vi "_readArray.vi"(8 "error in (no error)":errorcluster, 11 "JSONParser in":refnum<class "tJSONParser.lvclass">) -> (0 "error out":errorcluster, 2 "tBSONArray Out":refnum<class "tBSONArray.lvclass">, 3 "JSONParser out":refnum<class "tJSONParser.lvclass">)   [LabVIEW 2013, in "JSON.lvlib" / "tJSONParser.lvclass"]
doc: "Reads and validates an array value from a string : value pair. An error is returned if a comma is not followed by an array element."
uses:
  tJSONParser.lvclass
  BSON/BSONElements/tBSONArray/tBSONArray.lvclass
  BSON/tBSONElement/tBSONElement.lvclass
  tJSONParser.lvclass/tJSONParser.ctl
  _tokenType.ctl
  _error.ctl
  BSON/BSONElements/tBSONArray/setValue.vi
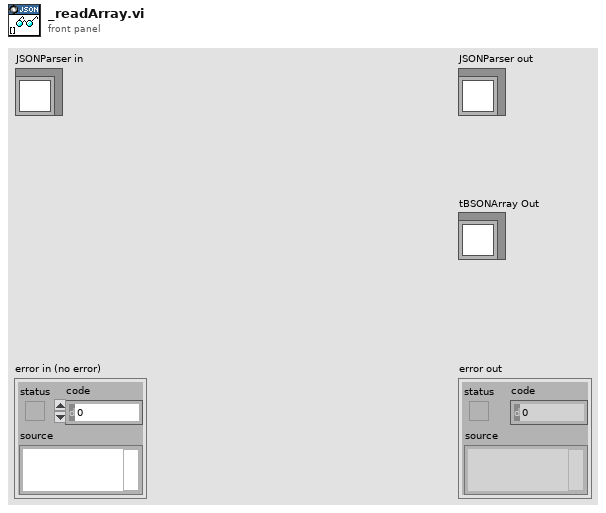
[diagram p1: front panel]
types:
  T1 = typedef "JSON.lvlib/tJSONParser.lvclass/_tokenType.ctl" = enum16{"Object Begin", "Object End", "Array Begin", "Array End", "String Delimeter", "Forward Slash", "Number", "Boolean", "Null", "Object Or Array Separator", "Pair Separator", "End Of File", "Asterisk", "Backward Slash", "Other"}
  T2 = typedef "JSON.lvlib/tJSONParser.lvclass/_error.ctl" = enum16{"Missing Object Open", "Missing Pair Separator", "Missing Object End Or Separator", "Missing Pair String", "Unexpected Token", "Missing Array End Or Separator", "Invalid Escape Sequence", "Unexpected End Of File", "Invalid Unicode", "Unexpected End Of Line", "Invalid Numerical Constant"}
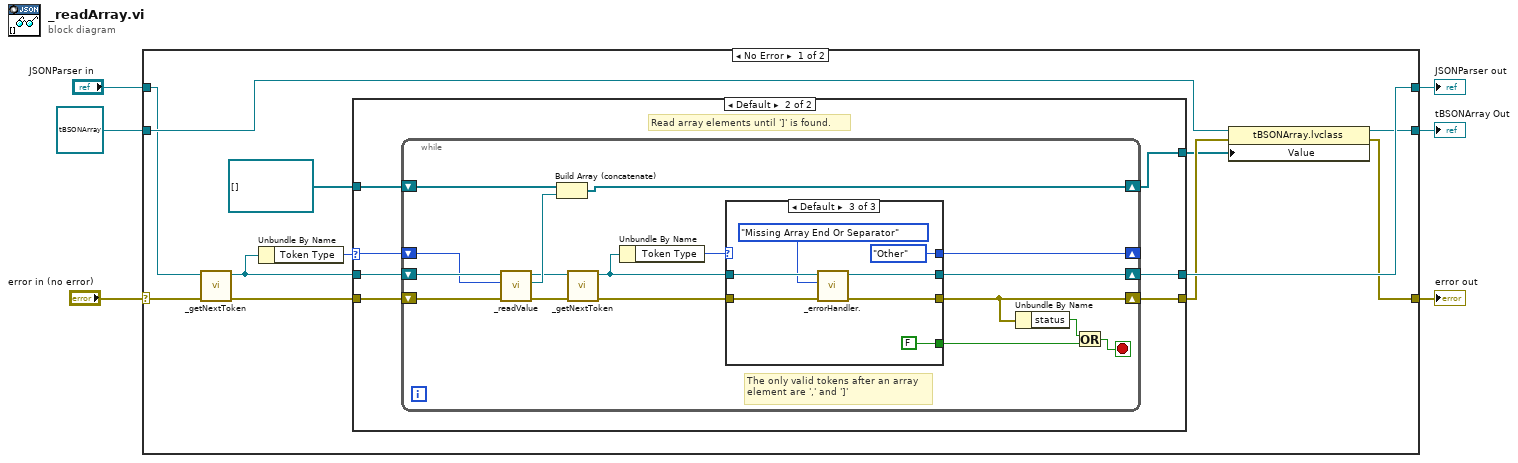
[diagram p0: block diagram]
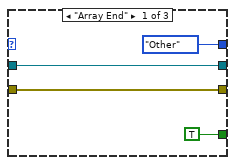
[diagram p3: hidden frame]
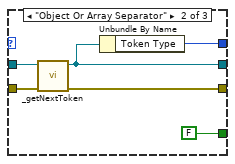
[diagram p4: hidden frame]
diagram:
  n1 = case shown="No Error" "error in (no error)" {
    selector: "error in (no error)" -> [w11 w65]
    tunnel: [w14 w65] -> w5
    tunnel: [w18 w64] -> w3
    tunnel: "JSONParser in" -> [w9 w64]
    tunnel: refnum<class "tBSONArray.lvclass"> refnum ("lvMongoDriver.lvlib:BSON.lvlib:tBSONArray.lvclass") -> [w17 w63]
    tunnel: [w16 w63] -> w1
    frame No Error {
      n2 = call "_getNextToken.vi"("error in (no error)"=w11, "JSON Parser In"=w9) -> ("error out"=w10:errorcluster, "JSON Parser Out"=w8:refnum<class "tJSONParser.lvclass">)  [unwired: 8 in]
      n3 = Unbundle By Name(w8) -> ("Token Type"=w7:T1)
      n4 = case shown="Default" w7 {
        selector: w7 -> [_ w22]
        tunnel: [w19 w28] -> w18
        tunnel: [w20 w27] -> w15
        tunnel: refnum<class "tBSONElement.lvclass">[] [] -> [w21 w26]
        tunnel: [w21 w25] -> w12
        tunnel: w8 -> [w19 w24]
        tunnel: w10 -> [w20 w23]
        frame "Array End" {
          # "Empty Array"
        }
        frame Default {
          # "Read array elements until ']' is found."
          n5 = while {
            shift-right: [w42] -> w27
            shift-left: w23 -> [w37]
            shift-right: [w43] -> w28
            shift-left: w24 -> [w38]
            shift-right: [w39] -> w25
            shift-left: w26 -> [w40]
            shift-right: [w29] -> _
            shift-left: w22 -> [w36]
            stop <- w44 stop-if-true
            # "The only valid tokens after an array\nelement are ',' and ']'"
            n6 = call "_readValue.vi"("error in (no error)"=w37, "Token Type"=w36, "JSONParser in"=w38) -> ("error out"=w34:errorcluster, "tBSONElement Out"=w35:refnum<class "tBSONElement.lvclass">, "JSONParser out"=w33:refnum<class "tJSONParser.lvclass">)  [unwired: 6 in]
            n7 = Build Array (concatenate)(w40, w35) -> (w39:refnum<class "tBSONElement.lvclass">[])
            n8 = call "_getNextToken.vi"("error in (no error)"=w34, "JSON Parser In"=w33) -> ("error out"=w32:errorcluster, "JSON Parser Out"=w30:refnum<class "tJSONParser.lvclass">)  [unwired: 8 in]
            n9 = Unbundle By Name(w30) -> ("Token Type"=w31:T1)
            n10 = case shown="Default" w31 {
              tunnel: w32 -> [w47 w54 w61]
              tunnel: w30 -> [w48 w53 w60]
              tunnel: [w47 w52 w59] -> w42
              tunnel: [w48 w51 w58] -> w43
              tunnel: [TRUE FALSE FALSE] -> w41
              tunnel: [_tokenType."Other" ("Token Type") w50 _tokenType."Other" ("Token Type")] -> w29
              frame "Array End" {
              }
              frame "Object Or Array Separator" {
                n11 = call "_getNextToken.vi"("error in (no error)"=w54, "JSON Parser In"=w53) -> ("error out"=w52:errorcluster, "JSON Parser Out"=w51:refnum<class "tJSONParser.lvclass">)  [unwired: 8 in]
                n12 = Unbundle By Name(w51) -> ("Token Type"=w50:T1)
              }
              frame Default {
                n13 = call "_errorHandler..vi"("error in (no error)"=w61, "Error Type"=_error."Missing Array End Or Separator", "JSON Parser In"=w60) -> ("error out"=w59:errorcluster, "JSON Parser Out"=w58:refnum<class "tJSONParser.lvclass">)  [unwired: 7 in]
              }
            }
            n14 = Unbundle By Name(w42) -> ("status"=w45:bool)
            n15 = Or(x=w45, y=w41) -> (x .or. y?=w44:bool)
          }
        }
      }
      n16 = property class="tBSONArray.lvclass"(reference=w17, error in=w15, "Value"=w12) -> (reference out=w16:refnum<class "tBSONArray.lvclass">, error out=w14:errorcluster)
    }
    frame Error {
    }
  }
  "error out" <- w5
  "JSONParser out" <- w3
  "tBSONArray Out" <- w1
